vi "Write Pulse driver.vi"(8 "error in (no error)":errorcluster, 10 "Pulse Driver.lvclass":refnum<class "Pulse Driver.lvclass">, 11 "Pulse Recorder in":refnum<class "Pulse Recorder Actor.lvclass">) -> (0 "error out":errorcluster, 3 "Pulse Recorder out":refnum<class "Pulse Recorder Actor.lvclass">)   [LabVIEW 2021, in "Pulse Recorder Actor.lvclass"]
uses:
  Pulse Recorder Actor.lvclass
  Pulse Recorder Actor.lvclass/Pulse Recorder Actor.ctl
  NHMFL_Core/Libraries/Instruments/Pulse Driver/Pulse Driver.lvclass
  C:/GitHub/NHMFL_Core/Libraries/Instruments/Instrument Driver/Instrument Driver.lvclass
  C:/GitHub/NHMFL_Core/Libraries/Instruments/Pulse Driver/Pulse Driver.lvclass
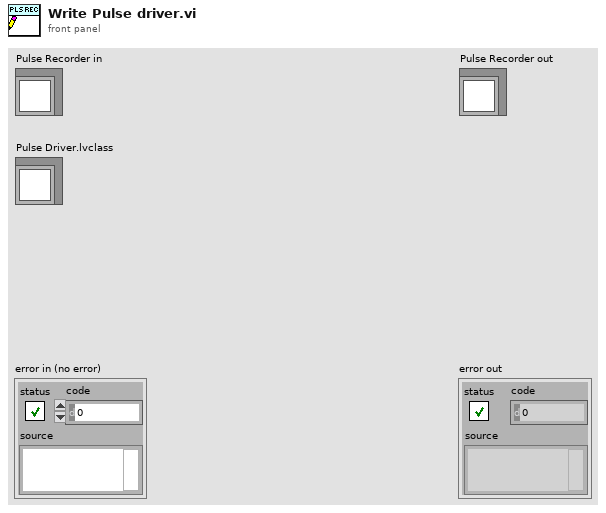
[diagram p1: front panel]
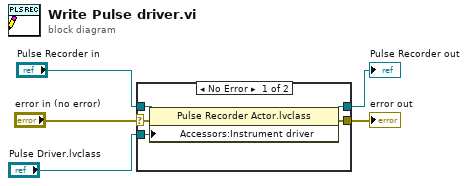
[diagram p0: block diagram]
diagram:
  n1 = case shown="No Error" "error in (no error)" {
    selector: "error in (no error)" -> [w7 w11]
    tunnel: [w6 w11] -> w4
    tunnel: [w8 w12] -> w2
    tunnel: "Pulse Recorder in" -> [w10 w12]
    tunnel: "Pulse Driver.lvclass" -> [w9 _]
    frame No Error {
      n2 = property class="Pulse Recorder Actor.lvclass"(reference=w10, error in=w7, "Accessors:Instrument driver"=w9) -> (reference out=w8:refnum<class "Pulse Recorder Actor.lvclass">, error out=w6:errorcluster)
    }
    frame Error {
    }
  }
  "error out" <- w4
  "Pulse Recorder out" <- w2
